vi "Homes.vi"() -> ()   [LabVIEW 2013]
panel:
  in  "Interposer Home":dbl=4.64
  in  "Comp Intake Home":dbl=4.64
  in  "Comp Arm Home":dbl=0.3
  in  "Winch Home":dbl=0.95
  in  "Intake Home":dbl=0.1
  in  "Arm Home":dbl=0.4
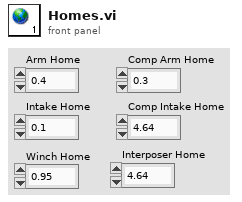
[diagram p1: front panel]
diagram:
